vi "SRV_Append to New Error Source String.vi"(0 "Filepath to append":path=path "XxXskipXxX", 1 "Append Call Chain (F)":bool, 5 "Message String to append":string, 11 "Error In (no error)":errorcluster, 12 "Previous Error In (no error)":errorcluster) -> (15 "error out":errorcluster)   [LabVIEW 2009]
doc: "Appends information to the error \"source\" string. This VI optionally appends:\n- Filepath\n- Message String\n- Call Chain\n\nWire <B>Previous Error In</B> to only append the above info if Previous Error In is False AND Error In is True. In other words 'Error In is a new error'.\n\n\nAuthor: Mike Schultz\n\n\nLogicPD, Inc\nwww.logicpd.com"
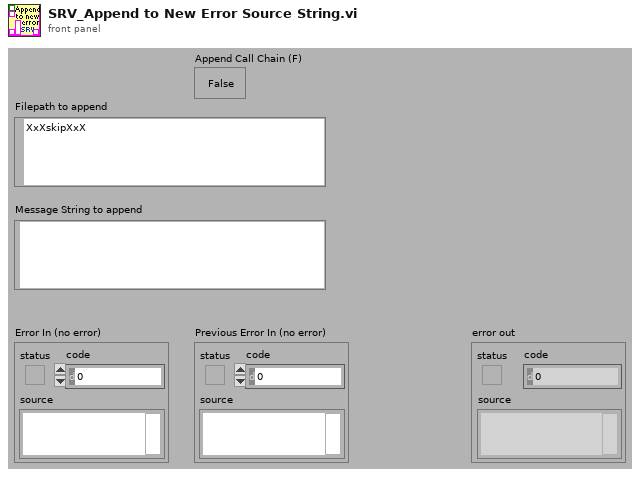
[diagram p1: front panel]
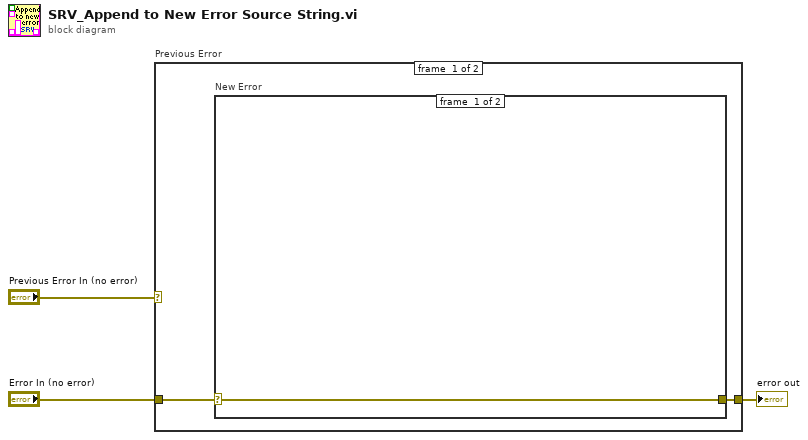
[diagram p0: block diagram]
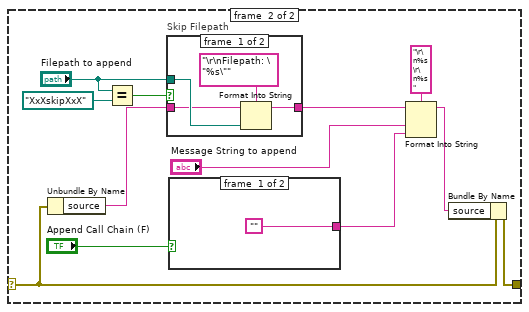
[diagram p2: hidden frame]
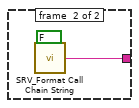
[diagram p3: hidden frame]
diagram:
  n1 = case "Previous Error" shown="No Error" "Previous Error In (no error)" {
    tunnel: "Error In (no error)" -> [w4 w27]
    tunnel: [w5 w27] -> w3
    frame #0 {
      n2 = case "New Error" shown="Error" w4 {
        selector: w4 -> [w6 w7]
        tunnel: [w6 w10] -> w5
        frame #0 {
        }
        frame #1 {
          n3 = Unbundle By Name(w7) -> ("source"=w15:string)
          n4 = Equal?(x="Filepath to append", y=path "XxXskipXxX" ("File Path to Append")) -> (x = y?=w16:bool)
          n5 = case "Skip Filepath" shown="False" w16 {
            tunnel: "Filepath to append" -> [w25 _]
            tunnel: w15 -> [w23 w26]
            tunnel: [w22 w26] -> w14
            frame #0 {
              n6 = Format Into String(format string="\r\nFilepath: \"%s\"" ("Format String"), initial string=w23, w25) -> (resulting string=w22:string)  [unwired: 1 in, 1 out]
            }
            frame #1 {
            }
          }
          n7 = case shown="True" "Append Call Chain (F)" {
            tunnel: ["" w21] -> w9
            frame #0 {
            }
            frame #1 {
              n8 = call "SRV_Format Call Chain String.vi"("Include This VI's Caller (T)"=FALSE) -> ("Formatted Call Chain String"=w21:string)  [unwired: 13 in, 1 out]
            }
          }
          n9 = Format Into String(format string="\r\n%s\r\n%s" ("Format String"), initial string=w14, "Message String to append", w9) -> (resulting string=w11:string)  [unwired: 1 in, 1 out]
          n10 = Bundle By Name(cluster=w7, "source"=w11) -> (w10:errorcluster)
        }
      }
    }
    frame #1 {
    }
  }
  "error out" <- w3
